vi "UV-VIS ShutDown.vi"(3 "error in (no error)":errorcluster, 5 "UV-VIS  in":refnum<class "CCD_camera.lvclass">) -> (0 "error out":errorcluster, 1 "DLL error code":u32, 2 "UV-VIS  out":refnum<class "CCD_camera.lvclass">)   [LabVIEW 2018, in "CCD_camera.lvclass"]
doc: "This function will close the AndorMCD[tm] system down.\n\n<B>Error code:</B>\nDRV_SUCCESS - System shut down.\n\n<B>NOTES:</B>\n<B>The temperature of the detector should be above zero degrees before shutting down the system.</B>"
uses:
  CCD_camera.lvclass
  C:/Users/Sergey Denisov/Documents/REPS/TRANCON/Classes/Detector/Detector.lvclass
  Detector.lvclass/Detector.ctl
  DLL/atmcd32d.dll
  Detector.lvclass
panel:
  out "DLL error code 2":u32
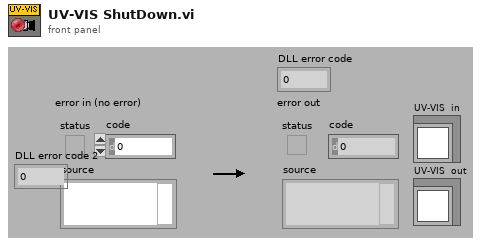
[diagram p1: front panel]
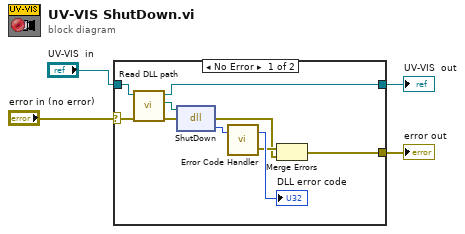
[diagram p0: block diagram]
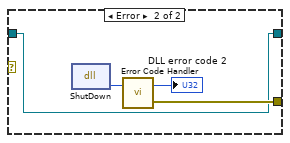
[diagram p2: hidden frame]
diagram:
  n1 = case shown="No Error" "error in (no error)" {
    selector: "error in (no error)" -> [w11 _]
    tunnel: [w6 w16] -> w3
    tunnel: [w5 w15] -> w2
    tunnel: "UV-VIS  in" -> [w12 w15]
    frame No Error {
      n2 = call "Read DLL path.vi"("error in (no error)"=w11, "Detector in"=w12) -> ("error out"=w9:errorcluster, "DLL path"=w8:path, "Detector out"=w5:refnum<class "CCD_camera.lvclass">)  [unwired: 7 in]
      n3 = dll-call lib="S:/TRANCON/DLL/atmcd32d.dll" fn="ShutDown"(path in=w8, error in=w9) -> (error out=w7:errorcluster, "return type"=w14:u32)  [unwired: 1 in, 1 out]
      n4 = call "Error Code Handler.vi"("DLL error code"=w14) -> ("error out"=w10:errorcluster, "dup DLL error code"=→"DLL error code":u32)  [unwired: 1 out]
      n5 = Merge Errors(w10, w7) -> (w6:errorcluster)
    }
    frame Error {
      n6 = dll-call lib="C:/Users/Sergey Denisov/Documents/REPS/TRANCON/DLL/Atmcd32d.dll" fn="ShutDown"() -> (w18:u32)  [unwired: 3 in, 2 out]
      n7 = call "Error Code Handler.vi"("DLL error code"=w18) -> ("error out"=w16:errorcluster, "dup DLL error code"=→"DLL error code 2":u32)  [unwired: 1 out]
    }
  }
  "error out" <- w3
  "UV-VIS  out" <- w2
